vi "LightSensor.vi"() -> ()   [LabVIEW 2012]
panel:
  out "Light":u8(slide) scale=0.0..255.0
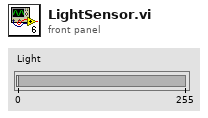
[diagram p1: front panel]
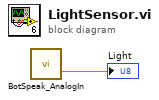
[diagram p0: block diagram]
diagram:
  n1 = call <userlib>:"BotSpeak_AnalogIn.vi"() -> ("voltage"=→"Light":dbl)  [unwired: 3 in, 1 out]
